vi "Get Waveform Data Size.vi"(8 "error in (no error)":errorcluster, 10 "Data String":u8[](array[numeric]), 11 "Type Descriptor":i16[](array[numeric])) -> (0 "error out":errorcluster, 2 "Data Size":i32)   [LabVIEW 2017, in "Composition.lvlib"]
doc: "Gets the data size of a waveform."
uses:
  Composition.lvlib
  ac5f3d2c-b102-4b6f-88c5-c2febea20318.vi
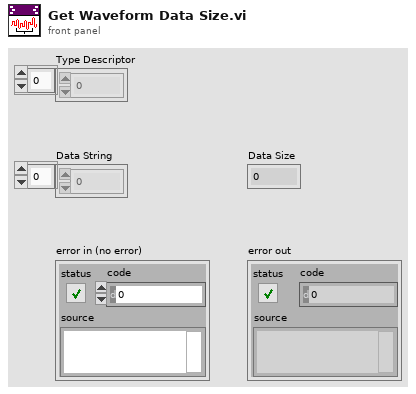
[diagram p1: front panel]
types:
  T1 = enum16{"0x00", "0x01", "I16", "DBL", "0x04", "SGL", "TimeStamp", "Digital Data", "Digital Waveform", "Dynamic Data", "EXT", "U8", "U16", "U32", "I8", "I32", "CSG", "CDB", "CXT", "I64", "U64"}
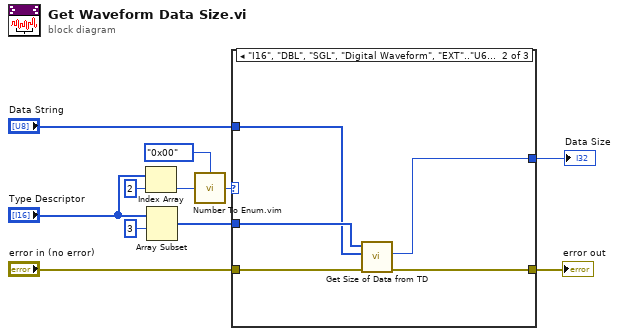
[diagram p0: block diagram]
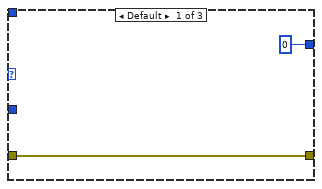
[diagram p2: hidden frame]
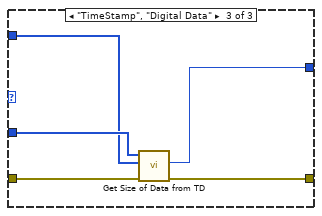
[diagram p3: hidden frame]
diagram:
  n1 = Index Array(array="Type Descriptor", index=2) -> (element=w10:i16)
  n2 = Array Subset(array="Type Descriptor", index=3) -> (w8:i16[])  [unwired: 1 in]
  n3 = call "Number To Enum.vim"("number"=w10, "enum type"=T1."0x00") -> ("number as enum"=w6:T1)
  n4 = case shown="\"I16\", \"DBL\", \"SGL\", \"Digital Waveform\", \"EXT\"..\"U64\"" w6 {
    tunnel: "Data String" -> [_ w17 w22]
    tunnel: [0 ("Size of Data") w14 w21] -> w1
    tunnel: w8 -> [_ w18 w23]
    tunnel: "error in (no error)" -> [w12 w16 w20]
    tunnel: [w12 w15 w19] -> w2
    frame Default {
    }
    frame "I16", "DBL", "SGL", "Digital Waveform", "EXT".."U64" {
      n5 = call "Get Size of Data from TD.vi"("error in (no error)"=w16, "Data String"=w17, "Type Descriptor"=w18) -> ("error out"=w15:errorcluster, "Size of Data"=w14:i32)  [unwired: 7 in]
    }
    frame "TimeStamp", "Digital Data" {
      n6 = call "Get Size of Data from TD.vi"("error in (no error)"=w20, "Data String"=w22, "Type Descriptor"=w23) -> ("error out"=w19:errorcluster, "Size of Data"=w21:i32)  [unwired: 7 in]
    }
  }
  "Data Size" <- w1
  "error out" <- w2
